vi "DB_GetMostFrequentID.vi"(8 "error in (no error)":errorcluster, 11 "SQLite Connection in":refnum<class "Connection.lvclass">) -> (0 "error out":errorcluster, 2 "Most Frequent ID":string, 3 "SQLite Connection out":refnum<class "Connection.lvclass">)   [LabVIEW 2020]
doc: "This VI outputs the most frequent car ID in the selected database using a basic SQL query."
uses:
  <vilib>/drjdpowell/SQLite Library/SQL Connection/Connection.lvclass
  <vilib>/drjdpowell/SQLite Library/SQL Statement/SQL Statement.lvclass/SQL Statement.ctl
  <vilib>/drjdpowell/SQLite Library/SQL Statement/Error Message.vi
  <vilib>/drjdpowell/SQLite Library/SQL Statement/Column String.vi
  <vilib>/drjdpowell/SQLite Library/SQL Statement/SQL Statement.lvclass
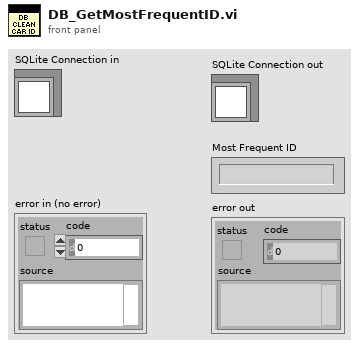
[diagram p1: front panel]
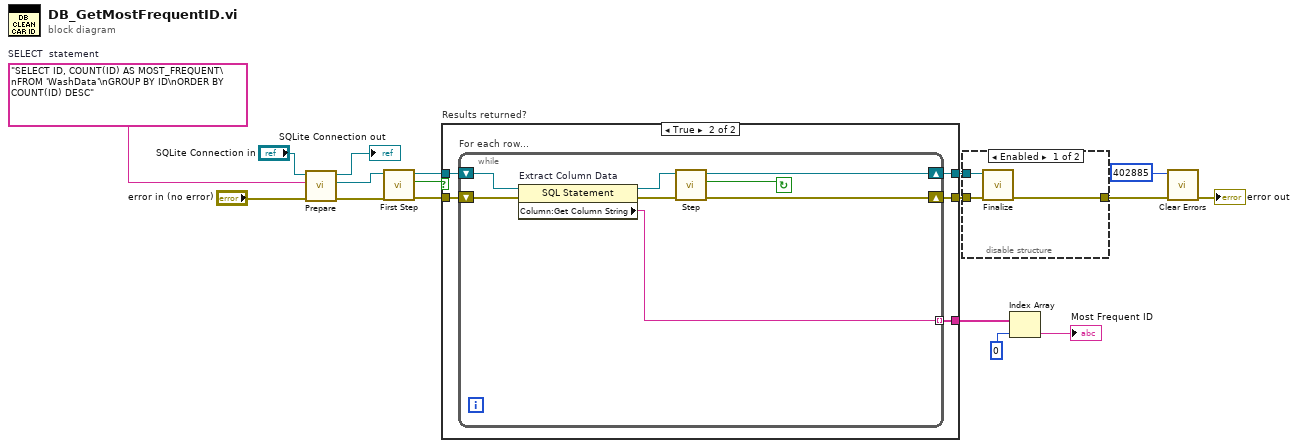
[diagram p0: block diagram]
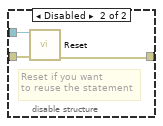
[diagram p2: hidden frame]
diagram:
  w15 = "SELECT ID, COUNT(ID) AS MOST_FREQUENT\nFROM 'WashData'\nGROUP BY ID\nORDER BY COUNT(ID) DESC"  # SELECT  statement
  n1 = call <vilib>:"Prepare.vi"("error in (no error)"="error in (no error)", "SQL"=w15, "SQLite Connection in"="SQLite Connection in") -> ("error out"=w11:errorcluster, "SQL Statement"=w10:refnum<class "SQL Statement.lvclass">, "SQLite Connection"=→"SQLite Connection out":refnum<class "Connection.lvclass">)  [unwired: 4 in, 2 out]
  n2 = call <vilib>:"First Step.vi"("error in (no error)"=w11, "SQL Statement in"=w10) -> ("error out"=w13:errorcluster, "Row returned"=w12:bool, "SQL Statement"=w14:refnum<class "SQL Statement.lvclass">)  [unwired: 7 in]
  n3 = case "Results returned?" shown="True" w12 {
    tunnel: [w19 w24] -> w16
    tunnel: [w18 w23] -> w17
    tunnel: w14 -> [w19 w22]
    tunnel: w13 -> [w18 w21]
    tunnel: [_ w20] -> w3
    frame False {
    }
    frame True {
      n4 = while "For each row..." {
        shift-right: [w31] -> w24
        shift-left: w22 -> [w28]
        shift-right: [w29] -> w23
        shift-left: w21 -> [w27]
        tunnel: [w25] -> w20 mode=indexing
        stop <- w26 continue-if-true
        n5 = property on="Extract Column Data" class="SQL Statement"(reference=w28, error in=w27) -> (reference out=w32:refnum<class "SQL Statement.lvclass">, error out=w30:errorcluster, "Column:Get Column String"=w25:string)
        n6 = call <vilib>:"Step.vi"("error in (no error)"=w30, "SQL Statement in"=w32) -> ("error out"=w29:errorcluster, "Row returned"=w26:bool, "SQL Statement"=w31:refnum<class "SQL Statement.lvclass">)  [unwired: 7 in]
      }
    }
  }
  n7 = disable-structure "Diagram Disable Structure" shown="Enabled" {
    disable-tunnel: w16 -> [w35 w38]
    disable-tunnel: w17 -> [w34 w37]
    disable-tunnel: [w33 w36] -> w6
    frame Enabled {
      n8 = call <vilib>:"Finalize.vi"("error in (no error)"=w34, "SQL Statement in"=w35) -> ("error out"=w33:errorcluster)  [unwired: 9 in]
    }
    frame Disabled {
      # "Reset if you want\nto reuse the statement"
      n9 = call <vilib>:"Reset.vi"("error in (no error)"=w37, "SQL Statement in"=w38) -> ("error out"=w36:errorcluster)  [unwired: 8 in, 1 out]
    }
  }
  n10 = Index Array(array=w3, index=0) -> (element=→"Most Frequent ID":string)
  n11 = call <vilib>:"Clear Errors.vi"("error in (no error)"=w6, "specific error code to clear (0: all)"=402885) -> ("error out"=→"error out":errorcluster)  [unwired: 4 in, 1 out]
